vi "Compass.vi"(10 "Delta X":dbl, 11 "Delta Y":dbl) -> (2 "Quadrant":i32, 3 "Angle":dbl)   [LabVIEW 2011]
uses:
  <vilib>/robotics/Controls/Compass Indicator/Compass Indicator.xctl
panel:
  out "Compass Indicator":dbl(xcontrol)
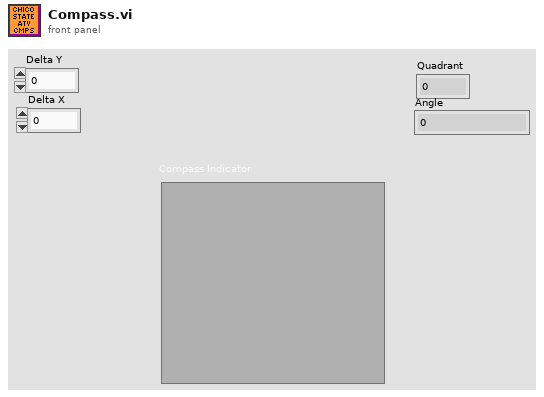
[diagram p1: front panel]
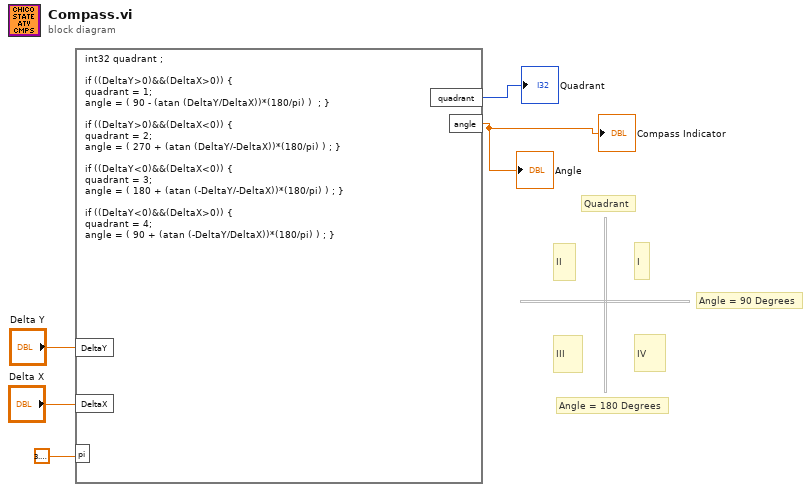
[diagram p0: block diagram]
diagram:
  # "Angle = 180 Degrees"
  # "Angle = 90 Degrees"
  # "IV"
  # "III"
  # "II"
  # "I"
  # "Quadrant"
  n1 = formula code="int32 quadrant ;\n\nif ((DeltaY>0)&&(DeltaX>0)) {\nquadrant = 1;\nangle = ( 90 - (atan (DeltaY/DeltaX))*(180/pi) )  ; }\n\nif ((DeltaY>0)&&(DeltaX<0)) {\nquadrant = 2;\nangle = ( 270 + (atan (DeltaY/-DeltaX))*(180/pi) ) ; }\n\nif ((DeltaY<0)&&(DeltaX<0)) {\nquadrant = 3;\nangle = ( 180 + (atan (-DeltaY/-DeltaX))*(180/pi) ) ; }\n\nif ((DeltaY<0)&&(DeltaX>0)) {\nquadrant = 4;\nangle = ( 90 + (atan (-DeltaY/DeltaX))*(180/pi) ) ; }"("DeltaY"="Delta Y", "DeltaX"="Delta X", "pi"=3.141592653589793) -> ("quadrant"=→"Quadrant":i32, "angle"=→"Angle" →"Compass Indicator":dbl)
